vi "justDW.vi"() -> ()   [LabVIEW 2019]
uses:
  <vilib>/eio/EIONode/EIONode.xnode
  <vilib>/rvi/eio/common/nirviEmuTemplateMethod_errors.vi
  <vilib>/eio/EIOPropertyNode/EIOPropertyNode.xnode
  <vilib>/rvi/eio/common/nirviEmuTemplatePropertyGet_errors.vi
  <vilib>/rvi/eio/common/nirviEmuTemplatePropertyGet_noerrors.vi
  <vilib>/rvi/eio/common/nirviEmuTemplatePropertySet_errors.vi
  <vilib>/rvi/eio/common/nirviEmuTemplatePropertySet_noerrors.vi
  <vilib>/rvi/DataTransferAndStorage/Container/XNode/niFpgaContainer.xnode
  <vilib>/rvi/FIFO/Fifo_Resource/nirvififoEmulationWrite.vi
  <vilib>/rvi/FIFO/Fifo_Resource/nirvififoEmulationRead.vi
  <vilib>/rvi/interface/RandomDataEmulation/nirviRandomDataFpgaReadWriteTemplate.vi
panel:
  in  "V_offset":sgl
  in  "Calibration":T1
  in  "Bias":sgl
  out "num of cycles":sgl
  in  "Fmax":sgl
  out "Fx out/Xcorr":sgl
  out "Xpot":sgl format="%.2f"
  in  "Temp":i8(ring) items=["Cold", "Warm", "Hot"]
  in  "cdfnorm":sgl
  out "Saveloop":u32
  in  "Enum":enum8{"No FB", "FB"}(ring)
  in  "MobX(px/V)":sgl
  in  "1/Xcali":sgl
  in  "Feedback parameters":T2
  in  "DX":sgl
  in  "DW":cluster{"xm":sgl, "Eb":sgl, "Tau":sgl, "dE":sgl}={"xm"=0.0, "Eb"=0.0, "Tau"=50.0, "dE"=0.0}
  in  "Xmean":sgl
  in  "Calibration ON/OFF":bool
  in  "Frequency":u32=100000
  in  "wait time":sgl=35.0
  in  "Triangle wave":T3={"signal offset_X"=5.0, "Scale X"=0.0, "signal offset_Y"=5.0, "Scale Y"=0.0, "Phase Shift"=30}
  in  "Xoffset":sgl
  in  "Yoffset":sgl
  in  "sum_offset":sgl
  in  "Normalize signal":bool=TRUE
  in  "FB Time":u8=5 caption="Feedback loop time"
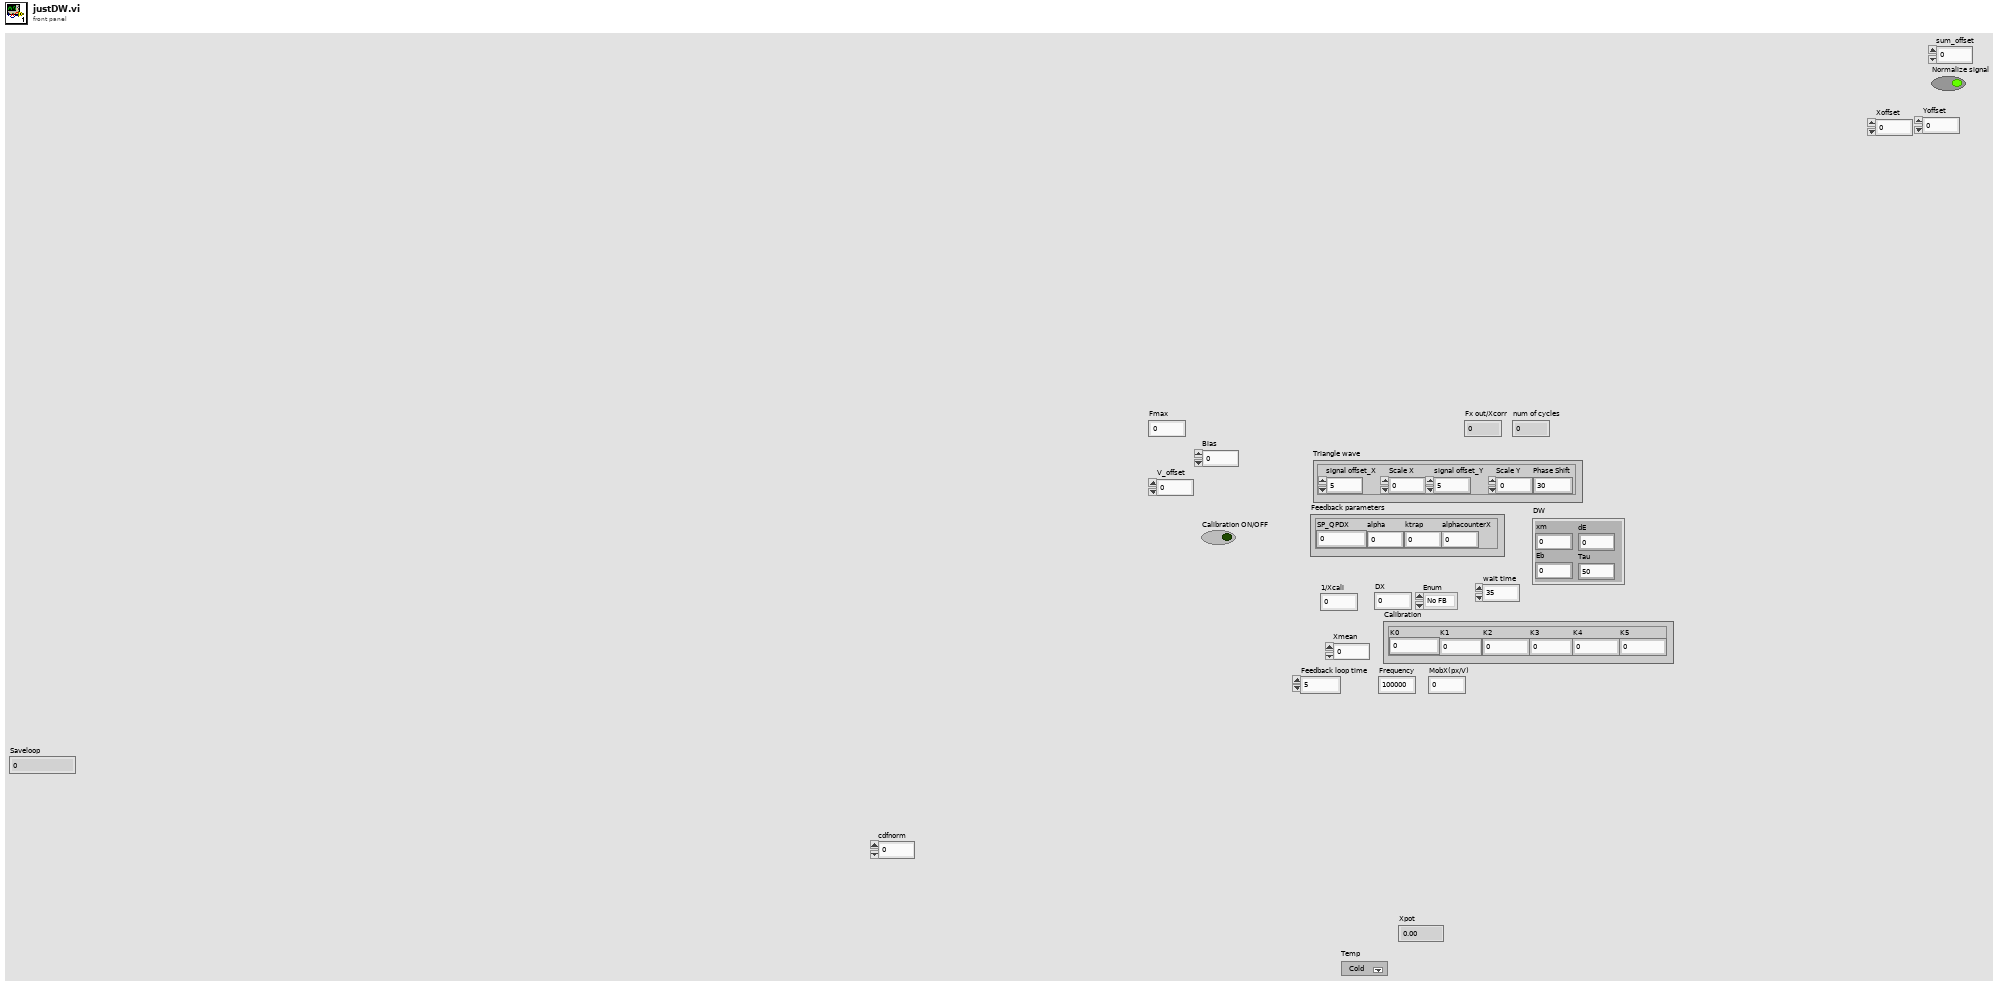
[diagram p1: front panel]
types:
  T1 = cluster{"K0":sgl, "K1":sgl, "K2":sgl, "K3":sgl, "K4":sgl, "K5":sgl}
  T2 = cluster{"SP_QPDX":sgl, "alpha":sgl, "ktrap":sgl, "alphacounterX":sgl}
  T3 = cluster{"signal offset_X":sgl, "Scale X":sgl, "signal offset_Y":sgl, "Scale Y":sgl, "Phase Shift":u32}
  T4 = enum8{"+/- 10 V", "+/- 5 V", "+/- 2 V", "+/- 1 V"}
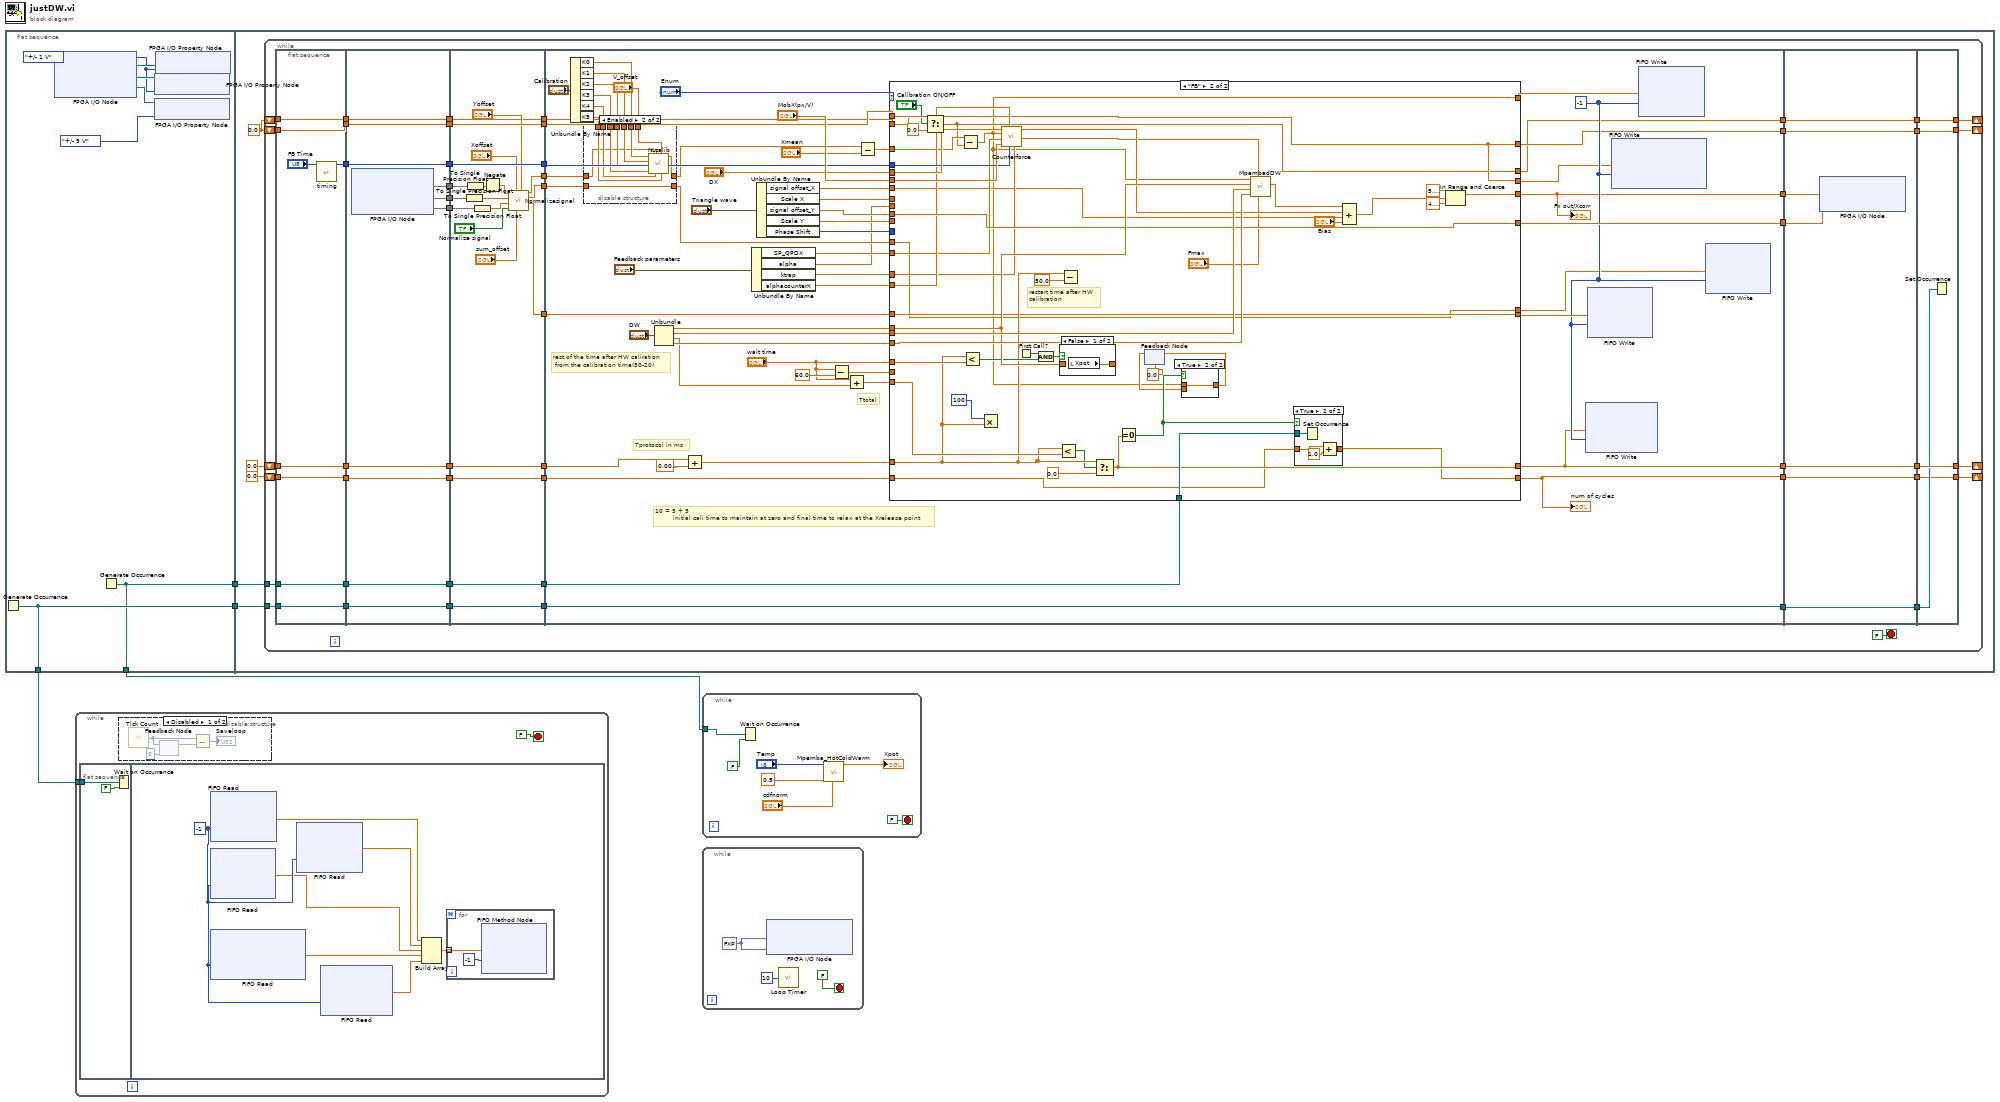
[diagram p0: block diagram]
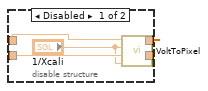
[diagram p2: hidden frame]
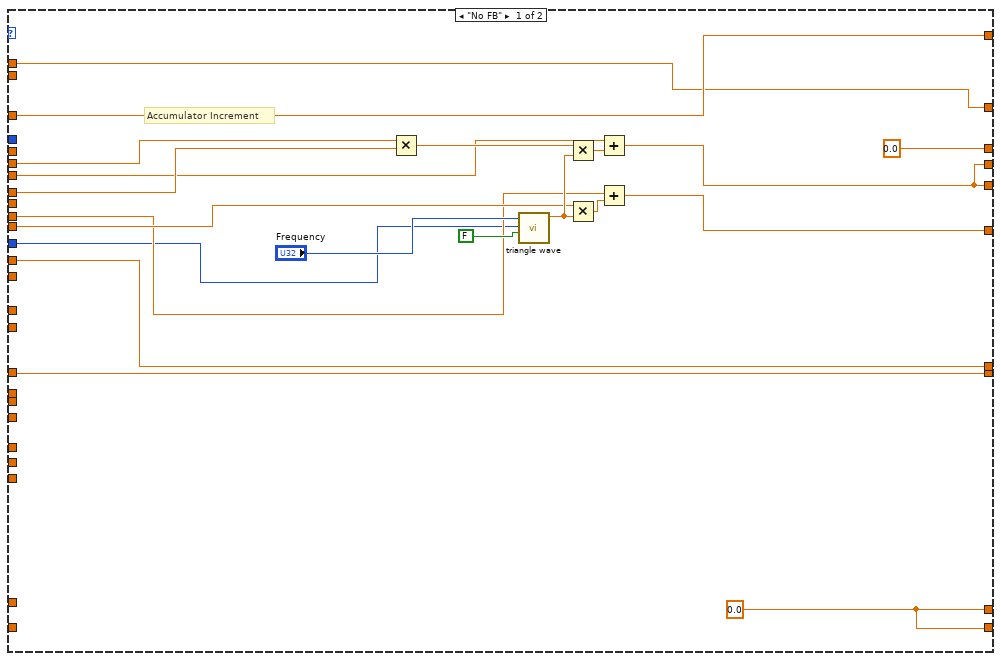
[diagram p3: hidden frame]
diagram:
  n1 = flat-sequence {
    tunnel: [w6] -> w2
    tunnel: [w5] -> w1
    tunnel: [w6] -> w4
    tunnel: [w5] -> w3
    tunnel: w2 -> [w16]
    tunnel: w1 -> [w15]
    frame #0 {
      w8 = T4."+/- 1 V" ("Voltage Range")
      n2 = Generate Occurrence() -> (w6:refnum<k4>)
      n3 = xnode "FPGA I/O Node"() -> ("FPGA I/O Out"=w11:refnum<k21>, "FPGA I/O Out"=w9:refnum<k21>, "FPGA I/O Out"=w10:refnum<k21>)  [unwired: 3 in, 3 out]
      n4 = Generate Occurrence() -> (w5:refnum<k4>)
      n5 = xnode "FPGA I/O Property Node"("FPGA I/O In"=w9, "Voltage Range"=w8) -> ()  [unwired: 1 out]
      n6 = xnode "FPGA I/O Property Node"("FPGA I/O In"=w10, "Voltage Range"=T4."+/- 5 V") -> ()  [unwired: 1 out]
      n7 = xnode "FPGA I/O Property Node"("FPGA I/O In"=w11, "Voltage Range"=w8) -> ()  [unwired: 1 out]
    }
    frame #1 {
      w12 = sgl 0.0
      n8 = while {
        tunnel: w16 -> [w47]
        shift-right: [w52] -> _
        shift-left: sgl 0.0 -> [w51]
        tunnel: w15 -> [w38]
        shift-right: [w35] -> _
        shift-left: w12 -> [w33]
        shift-right: [w28] -> _
        shift-left: sgl 0.0 ("f") -> [w26]
        shift-right: [w21] -> _
        shift-left: w12 -> [w20]
        stop <- FALSE ("stop") stop-if-true
        n9 = flat-sequence {
          tunnel: [w73] -> w55
          tunnel: w51 -> [w72]
          tunnel: [w72] -> w50
          tunnel: w47 -> [w71]
          tunnel: [w71] -> w46
          tunnel: [w70] -> w39
          tunnel: w38 -> [w70]
          tunnel: [w69] -> w34
          tunnel: w33 -> [w69]
          tunnel: [w68] -> w27
          tunnel: w26 -> [w68]
          tunnel: w20 -> [w67]
          tunnel: [w67] -> w19
          tunnel: [w84] -> w65
          tunnel: [w83] -> w63
          tunnel: [w82] -> w61
          tunnel: [w81] -> w56
          tunnel: w55 -> [w81]
          tunnel: w50 -> [w80]
          tunnel: [w80] -> w49
          tunnel: w46 -> [w79]
          tunnel: [w79] -> w45
          tunnel: [w78] -> w40
          tunnel: w39 -> [w78]
          tunnel: w34 -> [w77]
          tunnel: [w77] -> w31
          tunnel: w27 -> [w76]
          tunnel: [w76] -> w25
          tunnel: w19 -> [w75]
          tunnel: [w75] -> w18
          tunnel: w65 -> [w92]
          tunnel: [w104] -> w64
          tunnel: w63 -> [w91]
          tunnel: [w103] -> w62
          tunnel: w61 -> [w89]
          tunnel: [w102] -> w60
          tunnel: [w105] -> w57
          tunnel: w56 -> [w105]
          tunnel: w49 -> [w101]
          tunnel: [w101] -> w48
          tunnel: w45 -> [w100]
          tunnel: [w100] -> w44
          tunnel: [w99] -> w41
          tunnel: w40 -> [w99]
          tunnel: [w97] -> w32
          tunnel: w31 -> [w97]
          tunnel: w25 -> [w96]
          tunnel: [w96] -> w24
          tunnel: w18 -> [w87]
          tunnel: [w87] -> w17
          tunnel: w64 -> [w159]
          tunnel: w62 -> [w158]
          tunnel: w60 -> [w153]
          tunnel: [w114] -> w59
          tunnel: [w163] -> w58
          tunnel: w57 -> [w160]
          tunnel: [w133] -> w54
          tunnel: w48 -> [w155]
          tunnel: w44 -> [w146]
          tunnel: [w146] -> w42
          tunnel: w41 -> [w140]
          tunnel: [w135] -> w37
          tunnel: w32 -> [w134]
          tunnel: [w116] -> w30
          tunnel: w24 -> [w132]
          tunnel: [w118] -> w23
          tunnel: w17 -> [w117]
          tunnel: w58 -> [w260]
          tunnel: w59 -> [w261]
          tunnel: w54 -> [w259]
          tunnel: [w259] -> w53
          tunnel: [w258] -> w43
          tunnel: w42 -> [w258]
          tunnel: w37 -> [w257]
          tunnel: [w257] -> w36
          tunnel: w30 -> [w256]
          tunnel: [w256] -> w29
          tunnel: w23 -> [w255]
          tunnel: [w255] -> w22
          tunnel: w53 -> [w266]
          tunnel: [w266] -> w52
          tunnel: w43 -> [w265]
          tunnel: [w264] -> w35
          tunnel: w36 -> [w264]
          tunnel: w29 -> [w263]
          tunnel: [w263] -> w28
          tunnel: w22 -> [w262]
          tunnel: [w262] -> w21
          frame #0 {
            n10 = call "timing.vi"("Feedback loop time"="FB Time") -> ("Feedback Loop time"=w73:u32)  [unwired: 10 in]
          }
          frame #1 {
            n11 = xnode "FPGA I/O Node"() -> ("Connector1/AI2"=w84, "Connector1/AI4"=w83, "Connector1/AI5"=w82)  [unwired: 3 in, 3 out]
          }
          frame #2 {
            n12 = To Single Precision Float(number=w91) -> (single precision float=w90:sgl)
            n13 = To Single Precision Float(number=w92) -> (single precision float=w86:sgl)
            n14 = To Single Precision Float(number=w89) -> (single precision float=w88:sgl)
            n15 = Negate(x=w86) -> (-x=w85:sgl)
            n16 = call "Normalizesignal.vi"("Yoffset"="Yoffset", "sum_offset"="sum_offset", "Xoffset"="Xoffset", "Normalize signal"="Normalize signal", "Sum"=w88, "Y"=w90, "X"=w85) -> ("Sum"=w102:sgl, "Y"=w103:sgl, "X"=w104:sgl)  [unwired: 2 in]
          }
          frame #3 {
            w136 = -1 ("Timeout")
            # "rest of the time after HW caliration\n from the calibration time(50-20)"
            # "10 = 5 + 5\n         initial cali time to maintain at zero and final time to relax at the Xrelease point"
            # "Tprotocol in ms"
            # "Ttotal"
            n17 = Unbundle By Name("Calibration") -> ("K0"=w111:sgl, "K1"=w110:sgl, "K2"=w109:sgl, "K3"=w108:sgl, "K4"=w107:sgl, "K5"=w106:sgl)
            n18 = disable-structure shown="Enabled" {
              disable-tunnel: w159 -> [w168 w170]
              disable-tunnel: w158 -> [w167 w178]
              disable-tunnel: [w166 w178] -> w157
              disable-tunnel: [w165 w169] -> w143
              disable-tunnel: "V_offset" -> [_ w177]
              disable-tunnel: w111 -> [_ w176]
              disable-tunnel: w110 -> [_ w175]
              disable-tunnel: w109 -> [_ w174]
              disable-tunnel: w108 -> [_ w173]
              disable-tunnel: w107 -> [_ w172]
              disable-tunnel: w106 -> [_ w171]
              frame Disabled {
                n19 = call "VoltToPixel.vi"("1/(QPDY/px)"="1/Xcali", "Normalized Y"=w167, "1/(QPDX/px)"="1/Xcali", "Normalized X"=w168) -> ("Ypx"=w166:sgl, "Xpx"=w165:sgl)  [unwired: 6 in]
              }
              frame Enabled {
                n20 = call "NLcalib.vi"("K5"=w171, "V_offset"=w177, "K4"=w172, "Volt QPD"=w170, "K3"=w173, "K2"=w174, "K1"=w175, "K0"=w176) -> ("pixels"=w169:sgl)  [unwired: 3 in]
              }
            }
            n21 = Unbundle("DW") -> ("xm"=w141:sgl, "Eb"=w154:sgl, "Tau"=w120:sgl, "dE"=w148:sgl)
            n22 = Add(x=w155, y=sgl 0.01) -> (x+y=w147:sgl)
            n23 = Unbundle By Name("Feedback parameters") -> ("SP_QPDX"=w124:sgl, "alpha"=w121:sgl, "ktrap"=w122:sgl, "alphacounterX"=w123:sgl)
            n24 = Unbundle By Name("Triangle wave") -> ("signal offset_X"=w128:sgl, "Scale X"=w130:sgl, "signal offset_Y"=w127:sgl, "Scale Y"=w129:sgl, "Phase Shift"=w126:u32)
            n25 = Subtract(x="wait time", y=sgl 60.0) -> (x-y=w139:sgl)
            n26 = Add(x="wait time", y=w120) -> (x+y=w156:sgl)
            n27 = Subtract(x=w143, y="Xmean") -> (x-y=w151:sgl)
            n28 = case shown="\"FB\"" "Enum" {
              tunnel: w151 -> [w196 w204]
              tunnel: [w179 w221] -> w114
              tunnel: [w190 w220] -> w163
              tunnel: [w196 w202] -> w150
              tunnel: [w198 w209] -> w149
              tunnel: w153 -> [w198 w209]
              tunnel: w157 -> [w197 w206]
              tunnel: [w197 w206] -> w119
              tunnel: "MobX(px/V)" -> [w189 w242]
              tunnel: w160 -> [_ w225]
              tunnel: "DX" -> [_ w243]
              tunnel: w141 -> [_ w238]
              tunnel: w154 -> [_ w244]
              tunnel: w147 -> [_ w216]
              tunnel: w156 -> [_ w227]
              tunnel: [w181 w236] -> w133
              tunnel: w148 -> [_ w241]
              tunnel: w140 -> [_ w237]
              tunnel: "wait time" -> [_ w233]
              tunnel: w139 -> [_ _]
              tunnel: [w188 w212] -> w135
              tunnel: w134 -> [w188 w212]
              tunnel: [w181 w223] -> w116
              tunnel: w132 -> [_ w222]
              tunnel: w130 -> [w186 _]
              tunnel: w129 -> [w185 _]
              tunnel: w128 -> [w184 w205]
              tunnel: w127 -> [w183 w220]
              tunnel: w126 -> [w182 _]
              tunnel: w124 -> [_ w213]
              tunnel: w123 -> [_ w219]
              tunnel: w122 -> [_ w218]
              tunnel: w121 -> [_ _]
              tunnel: [sgl 0.0 ("f") w203] -> w118
              tunnel: w117 -> [_ w207]
              tunnel: [w179 w212] -> w115
              frame "No FB" {
                w181 = sgl 0.0 ("f")
                # "Accumulator Increment"
                n29 = Multiply(x=w189, y=w186) -> (x*y=w194:sgl)
                n30 = call "triangle wave.vi"("Reset Accumulator_TW"=FALSE, "phase shift"=w182, "Frequency"="Frequency") -> ("Tri wave out"=w191:sgl)  [unwired: 8 in]
                n31 = Multiply(x=w194, y=w191) -> (x*y=w193:sgl)
                n32 = Multiply(x=w185, y=w191) -> (x*y=w195:sgl)
                n33 = Add(x=w184, y=w193) -> (x+y=w179:sgl)
                n34 = Add(x=w183, y=w195) -> (x+y=w190:sgl)
              }
              frame "FB" {
                # "restart time after HW\ncalibration"
                n35 = Select(t=w207, s="Calibration ON/OFF", f=sgl 0.0) -> (s? t:f=w203:sgl)
                n36 = Subtract(x=w204, y=w203) -> (x-y=w202:sgl)
                n37 = Less?(x=w216, y=w233) -> (x < y?=w229:bool)
                n38 = Multiply(x=i16 100, y=w216) -> ()  [unwired: 1 out]
                n39 = call "Counterforce.vi"("ktrap"=w218, "Ts"=w225, "alphacounterX"=w219, "mobX(px/V)"=w242, "SP_X"=w213, "Xpx"=w202, "Dx"=w243) -> ("ktrap*mob"=w234:sgl, "counter Force"=w235:sgl)  [unwired: 2 in, 1 out]
                n40 = First Call?() -> (First Call?: T/F=w240:bool)
                n41 = And(x=w240, y=w229) -> (x .and. y?=w239:bool)
                n42 = Less?(x=w216, y=w227) -> (x < y?=w208:bool)
                n43 = case shown="False" w239 {
                  tunnel: [w253 w254] -> _
                  tunnel: w238 -> [_ w254]
                  frame False {
                    n44 = local read "Xpot"() -> (w253:sgl)
                  }
                  frame True {
                  }
                }
                n45 = Subtract(x=w216, y=sgl 50.0) -> ()  [unwired: 1 out]
                n46 = Select(t=w216, s=w208, f=sgl 0.0) -> (s? t:f=w236:sgl)
                n47 = Equal To 0?(x=w236) -> (x = 0?=w232:bool)
                n48 = feedback #1(sgl 0.0) -> (w230:sgl)
                n49 = case shown="True" w232 {
                  tunnel: w202 -> [_ w252]
                  tunnel: [w251 w252] -> w231
                  tunnel: w230 -> [w251 _]
                  frame False {
                  }
                  frame True {
                  }
                }
                n50 = feedback-in #1(w231) -> ()
                n51 = call "MpembadDW.vi"("Fmax"="Fmax", "ktrap*mob"=w234, "dE"=w241, "Eb"=w244, "Xm"=w238, "Xpos"=w202) -> ("DWvolt"=w199:sgl)  [unwired: 4 in, 1 out]
                n52 = case shown="True" w232 {
                  tunnel: w237 -> [_ w250]
                  tunnel: [w246 w249] -> w223
                  tunnel: w222 -> [w246 w248]
                  frame False {
                  }
                  frame True {
                    n53 = Set Occurrence(w250) -> ()
                    n54 = Add(x=w248, y=sgl 1.0) -> (x+y=w249:sgl)
                  }
                }
                n55 = Compound Arithmetic op=ADD(w199, w235, w205, "Bias") -> (w217:sgl)
                n56 = In Range and Coerce(upper limit=sgl 5.1, x=w217, lower limit=sgl 4.9) -> (coerced(x)=w221:sgl)  [unwired: 1 out]
              }
            }
            "Fx out/Xcorr" <- w114
            "num of cycles" <- w116
            n57 = xnode ("FIFO Write")("Element"=w133, "Timeout"=w136) -> ()  [unwired: 1 in, 2 out]
            n58 = xnode ("FIFO Write")("Element"=w149, "Timeout"=w136) -> ()  [unwired: 1 in, 2 out]
            n59 = xnode ("FIFO Write")("Element"=w115, "Timeout"=w136) -> ()  [unwired: 1 in, 2 out]
            n60 = xnode ("FIFO Write")("Element"=w150, "Timeout"=w136) -> ()  [unwired: 1 in, 2 out]
            n61 = xnode ("FIFO Write")("Element"=w119, "Timeout"=w136) -> ()  [unwired: 1 in, 2 out]
          }
          frame #4 {
            n62 = xnode "FPGA I/O Node"("Connector1/AO7"=w261, "Connector1/AO6"=w260) -> ()  [unwired: 2 in, 2 out]
          }
          frame #5 {
            n63 = Set Occurrence(w265) -> ()
          }
        }
      }
    }
  }
  n64 = while {
    tunnel: w4 -> [w267]
    stop <- FALSE stop-if-true
    n65 = flat-sequence {
      tunnel: w267 -> [w274]
      frame #0 {
        n66 = Wait on Occurrence(1:FALSE ("ignore previous (T)"), 2:w274) -> ()  [unwired: 1 in, 1 out]
      }
      frame #1 {
        w277 = -1 ("Timeout")
        n67 = xnode ("FIFO Read")("Timeout"=w277) -> ("Element"=w275:sgl)  [unwired: 1 in, 2 out]
        n68 = xnode ("FIFO Read")("Timeout"=w277) -> ("Element"=w278:sgl)  [unwired: 1 in, 2 out]
        n69 = xnode ("FIFO Read")("Timeout"=w277) -> ("Element"=w279:sgl)  [unwired: 1 in, 2 out]
        n70 = xnode ("FIFO Read")("Timeout"=w277) -> ("Element"=w276:sgl)  [unwired: 1 in, 2 out]
        n71 = xnode ("FIFO Read")("Timeout"=w277) -> ("Element"=w280:sgl)  [unwired: 1 in, 2 out]
        n72 = Build Array(w279, w276, w275, w278, w280) -> (w281:sgl[])
        n73 = for {
          tunnel: w281 -> [w283] mode=indexing
          n74 = xnode ("FIFO Method Node")("Element"=w283, "Timeout"=-1) -> ()  [unwired: 1 in, 2 out]
        }
      }
    }
    n75 = disable-structure shown="Disabled" {
      frame Disabled {
        n76 = call "Tick Count"() -> ("Tick Count(uSec)"=w272:u32)
        n77 = feedback #2(u32 0 ("Tick Count(uSec)")) -> (w271:u32)
        n78 = feedback-in #2(w272) -> ()
        n79 = Subtract(x=w272, y=w271) -> (x-y=→"Saveloop":u32)
      }
      frame Enabled {
      }
    }
  }
  n80 = while {
    stop <- FALSE stop-if-true
    w284 = fxp<+,8,3> 2.5 ("Connector1/AO2")
    n81 = xnode "FPGA I/O Node"("Connector1/AO0"=w284, "Connector1/AO4"=w284) -> ()  [unwired: 2 in, 2 out]
    n82 = call "Loop Timer"("Count(uSec)"=u8 10) -> ()  [unwired: 1 out]
  }
  n83 = while {
    tunnel: w3 -> [w292]
    stop <- FALSE ("stop") stop-if-true
    n84 = Wait on Occurrence(1:FALSE ("ignore previous (T)"), 2:w292) -> ()  [unwired: 1 in, 1 out]
    n85 = call "Mpemba_HotColdWarm.vi"("RN"="cdfnorm", "X0"=sgl 0.5, "Ring"="Temp") -> ("Xpot"=→"Xpot":sgl)  [unwired: 8 in]
  }
